vi "Example_OE2031&OE2041 Trig in.vi"() -> ()   [LabVIEW 2011]
panel:
  out "data_buffer":dbl[][](array[numeric])
  out "loss count":i32=-1
  out "cnt":u16
  in  "Ref_Source":u8(ring) items=["External", "Internal"]
  in  "Interval Count":u32=1 min=1 max=100000
  in  "选项卡控件":enum32{"选项卡 "}(tab)
  in  "Sweep Mode":u16(ring) items=["Linear", "Log"]
  in  "Start Frequency(Hz)":dbl=1000.0 min=1e-05 max=60000000.0 format="%#.3f"
  in  "Stop Frequency(Hz)":dbl=5000.0 min=1e-05 max=60000000.0 format="%#.3f"
  in  "Linear Step Frequency(Hz)":dbl=1000.0 min=1e-05 max=60000000.0 format="%#.3f"
  in  "Log Step Percent(%)":dbl=10.0 min=-100.0 max=100.0 format="%#.2f"
  in  "Step Time(ms)":i32=1000 min=50 max=100000
  in  "Sweep Run Mode":u16(ring) items=["Stop", "Singal", "Loop"]
  out "Group":u32
  in  "Sweep":u16(ring) items=["OFF", "ON"]
  in  "function":T1(ring)
  in  "Parameter Index":u16(ring) items=["X", "Y", "R", "θ", "Frequency", "XD1", "YD1", "RD1", "θD1", "XD2", "YD2", "RD2", "θD2", "XD3", "YD3", "RD3", "θD3", "X_Noise", "Y_Noise", "AUXADC1", "AUXADC2", "AUXADC3", "AUXADC4"]
  out "Wave":dbl(graph)
  in  "IP Address":string="192.168.1.10"
  in  "Timeout":u32=100
  in  "Port":u32=10001
  in  "Connect":bool
  in  "Trig Mode":u8(ring) items=["Internal", "Ext_Rissing_Edge", "Ext_Falling_Edge", "Ext_High_Level", "Ext_Low_Level"]
  out "Error out":errorcluster caption="error out"
  in  "Remote Mode":u16(ring) items=["USB"=0, "Ethernet"=3]
  in  "VISA resource name":refnum<visa-resource-name>
  # "Tel          :   +86-020-84133345\nWebsite  :   www.ssi-instrument.com\nE-mail     :   support@si-instrument.com"
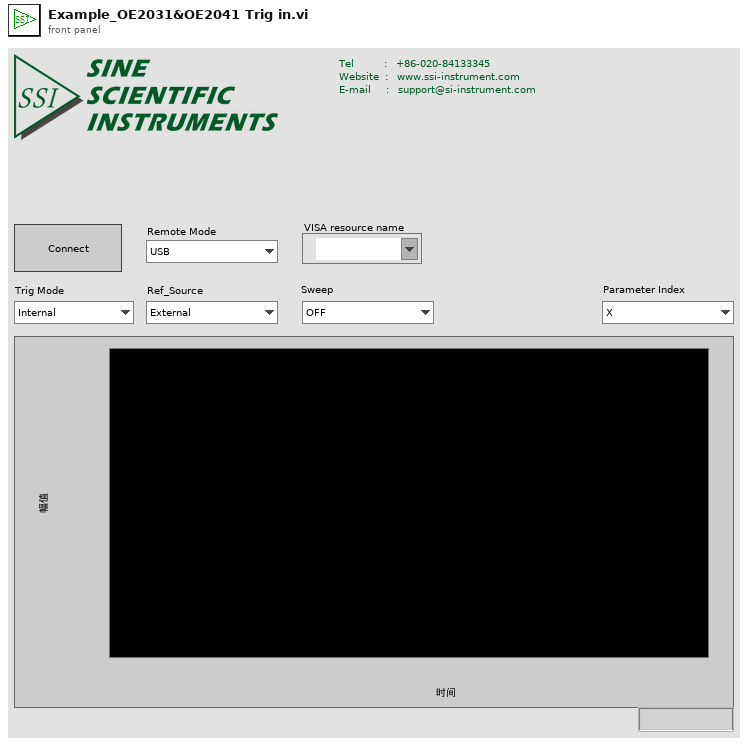
[diagram p1: front panel]
types:
  T1 = enum16{"initial", "Trig In Type", "Sample", "Ext_Sweep_Trig In", "Int_Sweep_Trig In"}
  T2 = enum8{"Enabled", "Disabled", "Disabled and Grayed Out"}
  T3 = cluster{"Port":u32, "Timeout":u32, "IP Address":string}
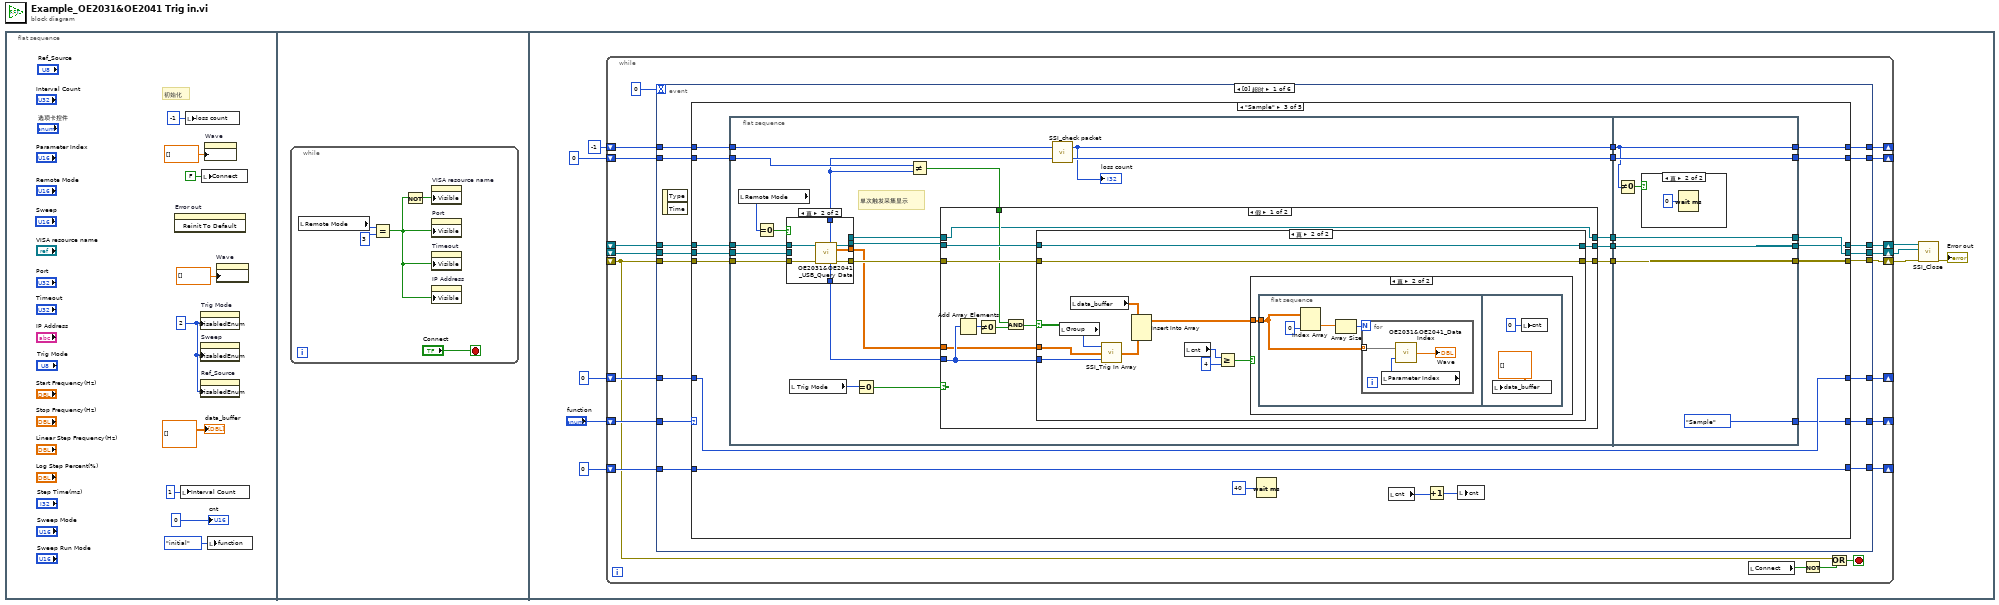
[diagram p0: block diagram]
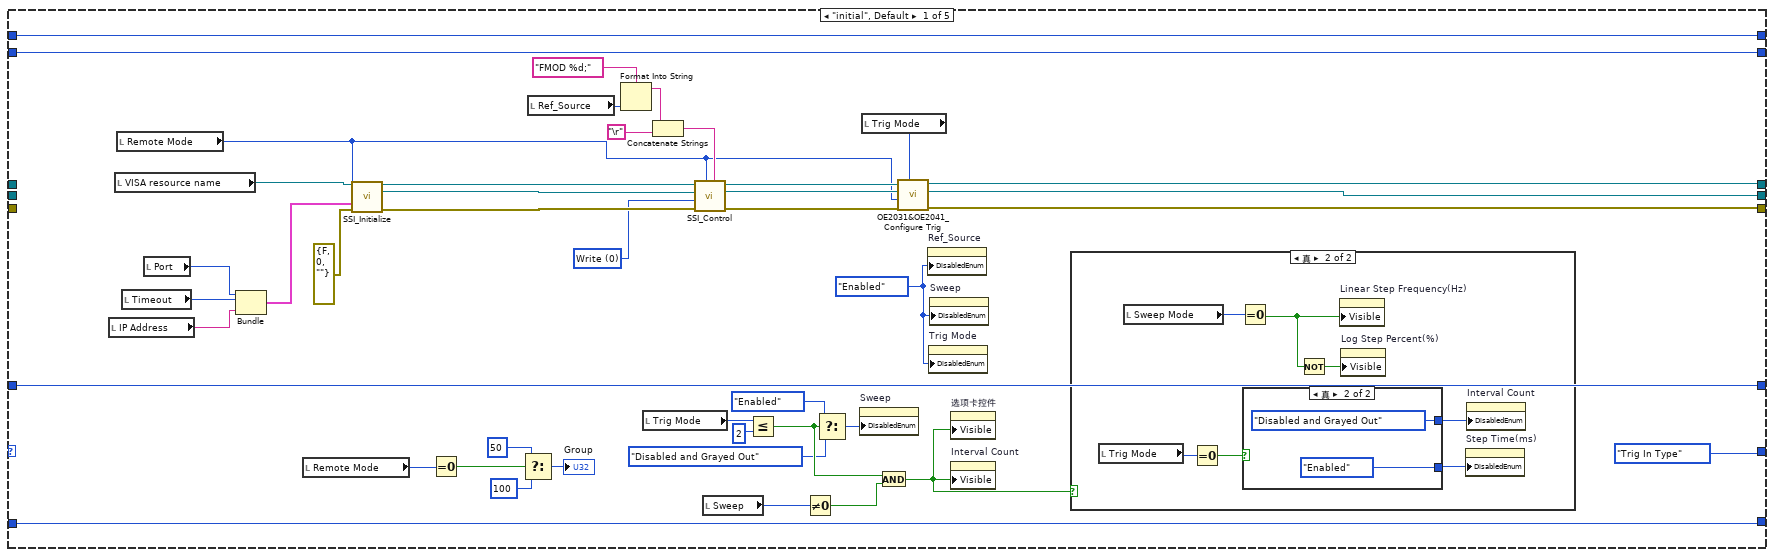
[diagram p2: hidden frame]
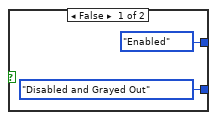
[diagram p4: hidden frame]
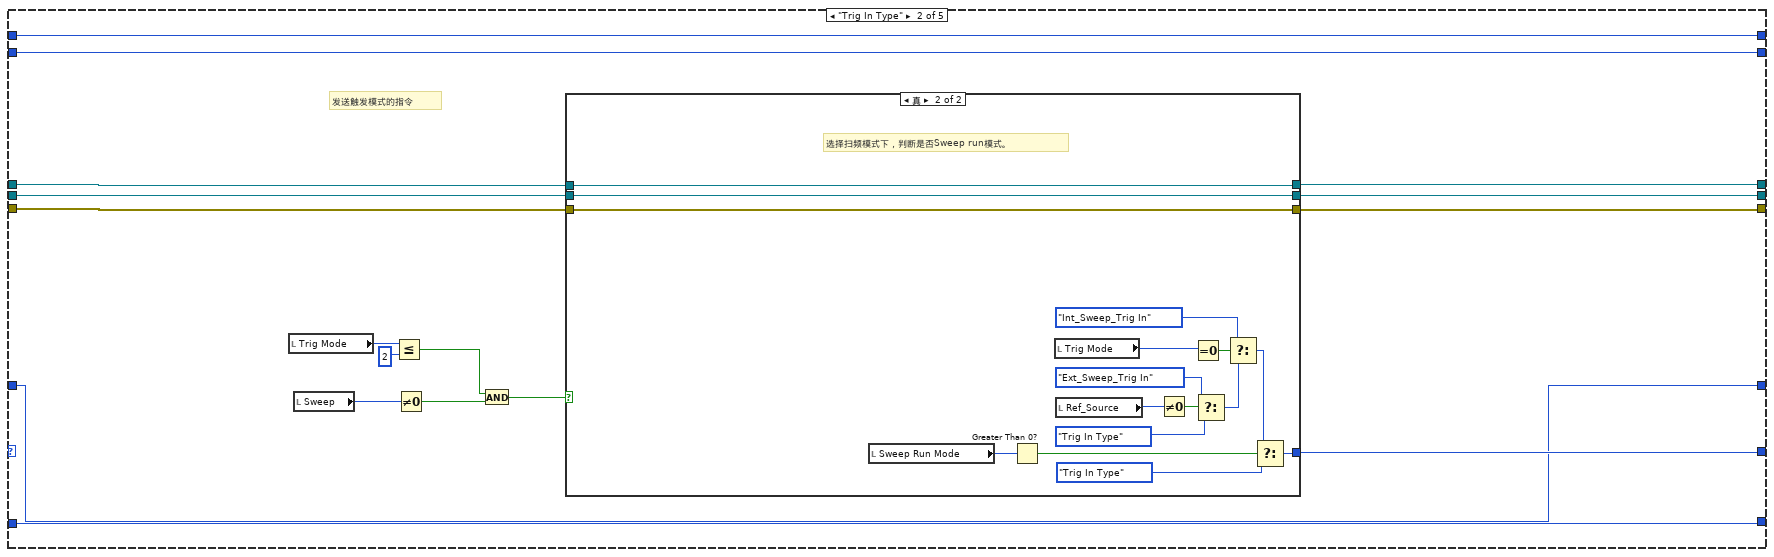
[diagram p5: hidden frame]
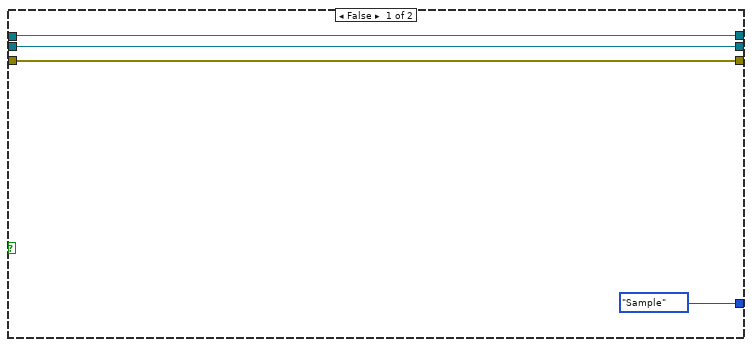
[diagram p6: hidden frame]
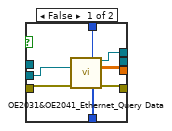
[diagram p7: hidden frame]
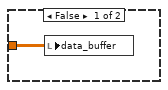
[diagram p9: hidden frame]
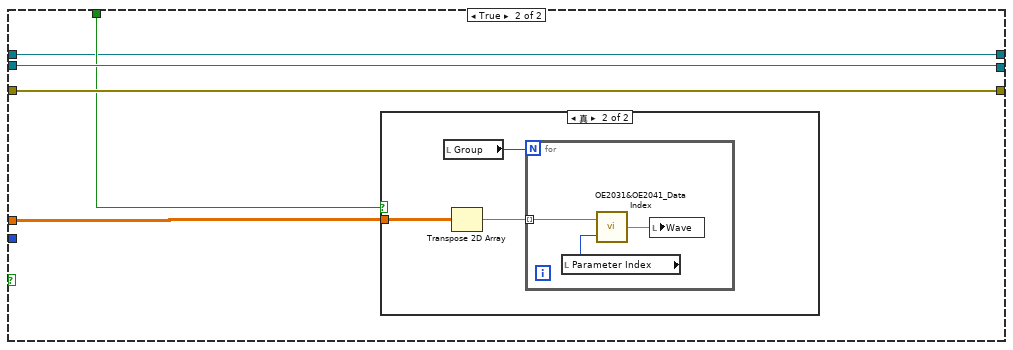
[diagram p10: hidden frame]
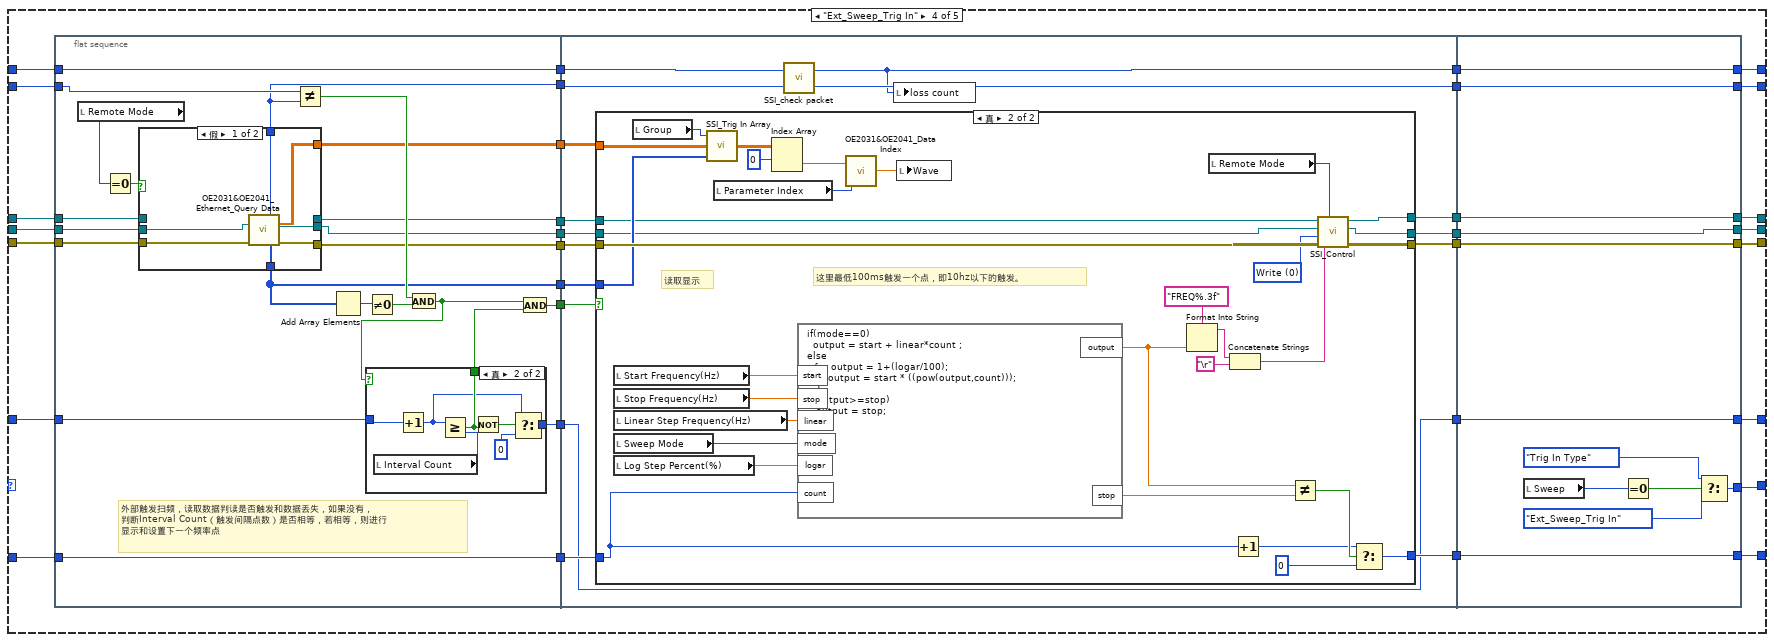
[diagram p13: hidden frame]
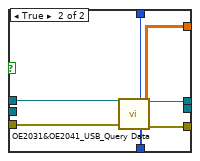
[diagram p14: hidden frame]
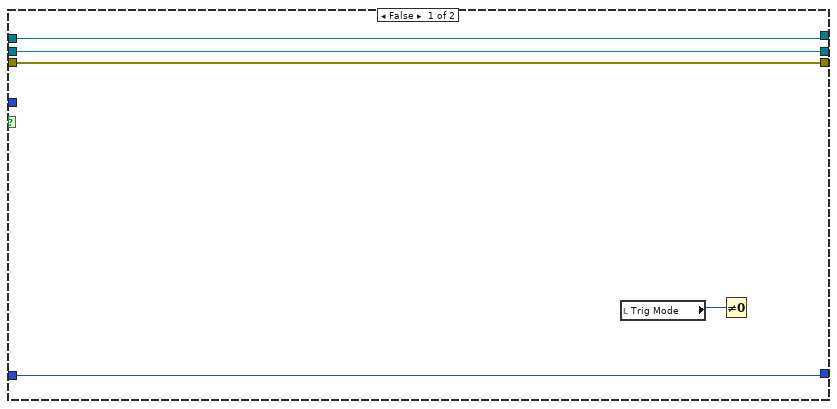
[diagram p16: hidden frame]
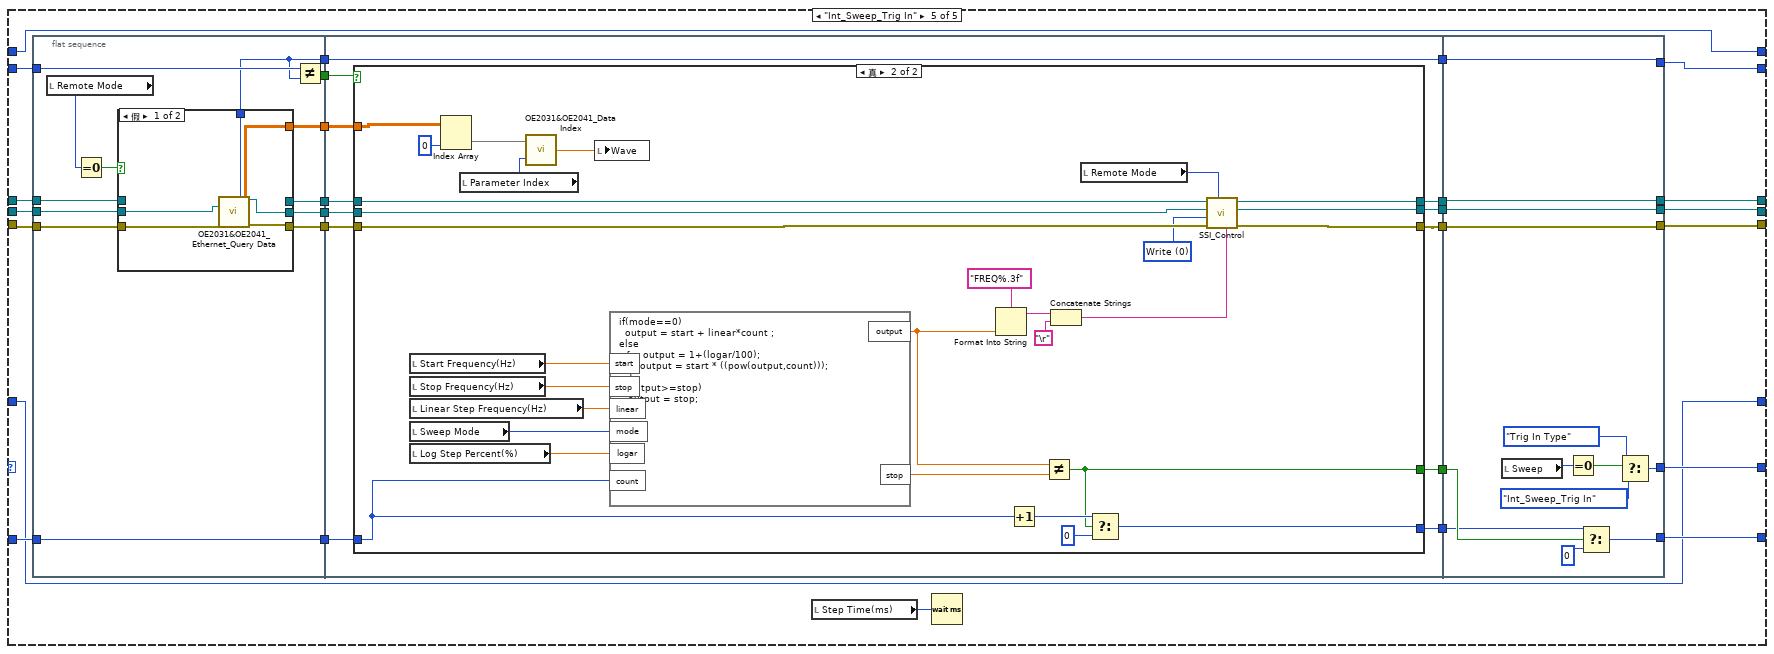
[diagram p17: hidden frame]
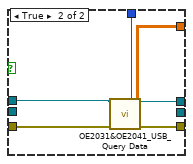
[diagram p18: hidden frame]
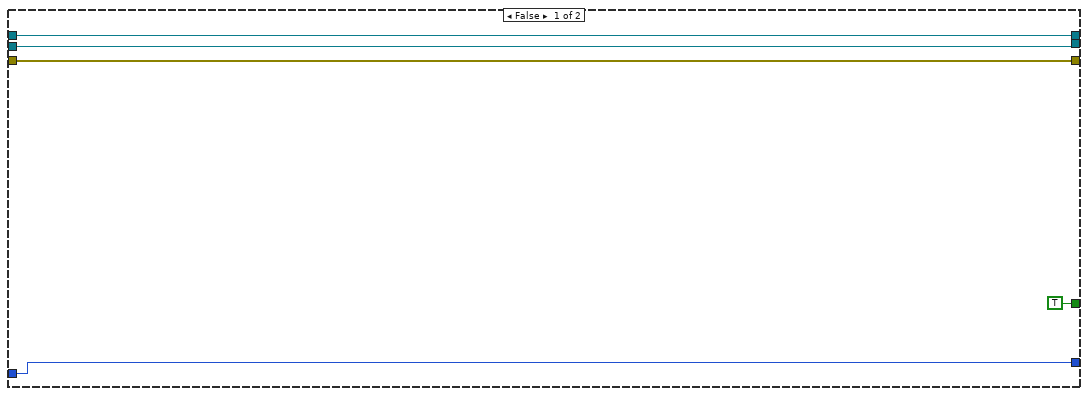
[diagram p19: hidden frame]
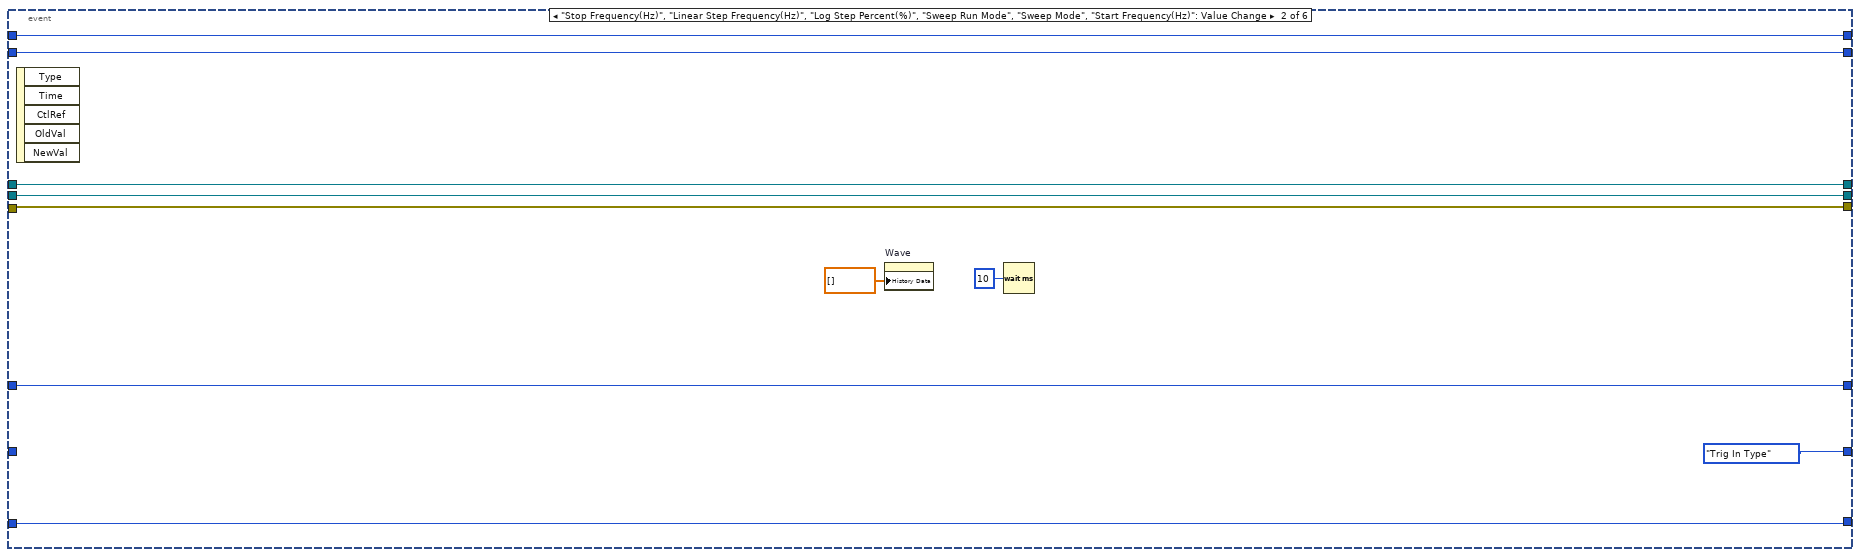
[diagram p20: hidden frame]
diagram:
  n1 = flat-sequence {
    frame #0 {
      w2 = 2
      # "初始化"
      n2 = invoke on="Error out" class="Clust (严格)" method="Reinit To Default"() -> ()  [unwired: 3 in, 3 out]
      n3 = local write "Interval Count"(u32 1 ("Interval Count")) -> ()
      n4 = local write "loss count"(-1 ("loss count")) -> ()
      n5 = property on="Trig Mode" class="Ring (严格)"("DisabledEnum"=w2) -> ()  [unwired: 2 in, 2 out]
      n6 = property on="Sweep" class="Ring (严格)"("DisabledEnum"=w2) -> ()  [unwired: 2 in, 2 out]
      n7 = property on="Ref_Source" class="Ring (严格)"("DisabledEnum"=w2) -> ()  [unwired: 2 in, 2 out]
      n8 = local write "Connect"(FALSE ("Connect")) -> ()
      n9 = property on="Wave" class="WFChart (严格)"("History Data"=dbl[] [] ("历史数据")) -> ()  [unwired: 2 in, 2 out]
      n10 = local write "function"(T1."initial" ("function")) -> ()
      n11 = property on="Wave" class="WFChart (严格)"("History Data"=dbl[] [] ("历史数据")) -> ()  [unwired: 2 in, 2 out]
      "data_buffer" <- dbl[][] []
      "cnt" <- 0
    }
    frame #1 {
      n12 = while {
        stop <- "Connect" stop-if-true
        n13 = local read "Remote Mode"() -> (w13:u16)
        n14 = Equal?(x=w13, y=u16 3) -> (x = y?=w11:bool)
        n15 = Not(x=w11) -> (.not. x?=w10:bool)
        n16 = property on="VISA resource name" class="VISAName"("Visible"=w10) -> ()  [unwired: 2 in, 2 out]
        n17 = property on="Port" class="DigNum (严格)"("Visible"=w11) -> ()  [unwired: 2 in, 2 out]
        n18 = property on="Timeout" class="DigNum (严格)"("Visible"=w11) -> ()  [unwired: 2 in, 2 out]
        n19 = property on="IP Address" class="Str"("Visible"=w11) -> ()  [unwired: 2 in, 2 out]
      }
    }
    frame #2 {
      n20 = while {
        shift-right: [w38] -> _
        shift-left: "function" -> [w39]
        shift-right: [w36] -> _
        shift-left: 0 ("f") -> [w37]
        shift-right: [w33] -> _
        shift-left: 0 -> [w34]
        shift-right: [w30] -> _
        shift-left: 0 -> [w31]
        shift-right: [w27] -> w17
        shift-left: _ -> [w41]
        shift-right: [w40] -> w22
        shift-left: _ -> [w29]
        shift-right: [w28] -> w18
        shift-left: _ -> [w26]
        shift-right: [w24] -> _
        shift-left: -1 ("loss count") -> [w25]
        stop <- w42 stop-if-true
        n21 = event shown="[0] 超时" {
          selector: _ -> [_ _ _ _ _ _]
          dyn-events: _ -> [_ _ _ _ _ _]
          timeout: 0 -> [_ _ _ _ _ _]
          tunnel: w41 -> [w59 w516 w528 w547 w573 w592]
          tunnel: [w58 w516 w528 w542 w572 w592] -> w27
          tunnel: [w57 w514 w527 w544 w575 w593] -> w40
          tunnel: w29 -> [w56 w514 w527 w549 w576 w593]
          tunnel: w39 -> [w55 _ _ _ w579 _]
          tunnel: [w54 T1."Trig In Type" ("function") T1."Trig In Type" ("function") T1."Trig In Type" ("function") w579 T1."Trig In Type" ("function")] -> w38
          tunnel: w37 -> [w53 w520 w530 w554 w580 w588]
          tunnel: [w52 w520 w530 w554 w580 w588] -> w36
          tunnel: w34 -> [w51 w518 w525 w552 w577 w590]
          tunnel: [w50 w518 w525 w552 w577 w590] -> w33
          tunnel: w31 -> [w49 w511 w524 w553 w578 w587]
          tunnel: [w48 w511 w524 w553 w578 w587] -> w30
          tunnel: [w47 w515 w522 w543 w571 w591] -> w28
          tunnel: w26 -> [w46 w515 w522 w548 w574 w591]
          tunnel: w25 -> [w45 w517 w521 w531 w566 w589]
          tunnel: [w44 w517 w521 w531 w566 w589] -> w24
          event Timeout {
            n22 = event-data() -> ()  [unwired: 1 in, 2 out]
            n23 = case shown="\"Sample\"" w55 {
              tunnel: w59 -> [_ w130 w170 w291 w411]
              tunnel: w56 -> [_ w128 w169 w290 w410]
              tunnel: [w81 w129 w153 w287 w424] -> w58
              tunnel: [w79 w127 w161 w288 w423] -> w57
              tunnel: [T1."Trig In Type" ("function") w126 w167 w276 w421] -> w54
              tunnel: w53 -> [w96 w125 w171 w289 w422]
              tunnel: [w96 w125 w171 w286 w420] -> w52
              tunnel: w51 -> [w94 w124 w166 w285 w426]
              tunnel: [w94 w124 w164 w284 w425] -> w50
              tunnel: w49 -> [w95 w123 w168 w271 w419]
              tunnel: [w95 w123 w168 w268 w419] -> w48
              tunnel: [w80 w115 w154 w264 w402] -> w47
              tunnel: w46 -> [_ w116 w156 w267 w406]
              tunnel: w45 -> [w61 w114 w159 w263 w401]
              tunnel: [w61 w114 w152 w260 w401] -> w44
              frame "initial", Default {
                w60 = T2."Enabled" ("禁用")
                w73 = u16 0 items=["Write", "Read"] ("Control")
                n24 = local read "IP Address"() -> (w76:string)
                n25 = local read "VISA resource name"() -> (w82:refnum<visa-resource-name>)
                n26 = local read "Remote Mode"() -> (w62:u16)
                n27 = local read "Timeout"() -> (w77:u32)
                n28 = local read "Port"() -> (w78:u32)
                n29 = Bundle("Port"=w78, "Timeout"=w77, "IP Address"=w76) -> (w75:T3)  [unwired: 1 in]
                n30 = local read "Remote Mode"() -> (w102:u16)
                n31 = call "SSI_Initialize.vi"("VISA resource name"=w82, "Remote Mode"=w62, "Ethernet"=w75, "error in (no error)"=errorcluster {"status"=FALSE, "code"=0, "source"=""}) -> ("VISA resource name out"=w86:refnum<visa-resource-name>, "connection ID(Ethernet)"=w87:refnum<k5>, "error out"=w83:errorcluster)  [unwired: 9 in]
                n32 = Equal To 0?(x=w102) -> (x = 0?=w98:bool)
                n33 = Select(t=50, s=w98, f=100) -> (s? t:f=→"Group":i32)
                n34 = local read "Ref_Source"() -> (w92:u8)
                n35 = Format Into String(format string="FMOD %d;" ("格式字符串"), w92) -> (resulting string=w93:string)  [unwired: 2 in, 1 out]
                n36 = local read "Trig Mode"() -> (w68:u8)
                n37 = Concatenate Strings(w93, "\r") -> (w72:string)
                n38 = call "SSI_Control.vi"("Write Buffer"=w72, "Remote Mode"=w62, "Error in (no error)"=w83, "Control"=w73, "Connection ID in"=w87, "VISA resource name"=w86) -> ("Error out"=w84:errorcluster, "Connection ID out"=w85:refnum<k5>, "VISA resource  out"=w88:refnum<visa-resource-name>)  [unwired: 2 in, 1 out]
                n39 = local read "Sweep"() -> (w69:u16)
                n40 = Less Or Equal?(x=w68, y=u8 2) -> (x <= y?=w70:bool)
                n41 = Not Equal To 0?(x=w69) -> (x != 0?=w71:bool)
                n42 = Select(t=T2."Enabled" ("禁用"), s=w70, f=T2."Disabled and Grayed Out") -> (s? t:f=w65:T2)
                n43 = property on="Sweep" class="Ring (严格)"("DisabledEnum"=w65) -> ()  [unwired: 2 in, 2 out]
                n44 = local read "Trig Mode"() -> (w89:u8)
                n45 = And(x=w70, y=w71) -> (x .and. y?=w63:bool)
                n46 = call "OE2031&OE2041_Configure Trig.vi"("Trig Mode"=w89, "Error in (no error)"=w84, "Remote Mode"=w62, "Connection ID in"=w85, "VISA resource name"=w88) -> ("Error out"=w79:errorcluster, "Connection ID out"=w80:refnum<k5>, "VISA resource  out"=w81:refnum<visa-resource-name>)  [unwired: 3 in, 1 out]
                n47 = property on="Ref_Source" class="Ring (严格)"("DisabledEnum"=w60) -> ()  [unwired: 2 in, 2 out]
                n48 = property on="Trig Mode" class="Ring (严格)"("DisabledEnum"=w60) -> ()  [unwired: 2 in, 2 out]
                n49 = property on="Sweep" class="Ring (严格)"("DisabledEnum"=w60) -> ()  [unwired: 2 in, 2 out]
                n50 = property on="选项卡控件" class="TabCtl (严格)"("Visible"=w63) -> ()  [unwired: 2 in, 2 out]
                n51 = property on="Interval Count" class="DigNum (严格)"("Visible"=w63) -> ()  [unwired: 2 in, 2 out]
                n52 = case shown="真" w63 {
                  frame False {
                  }
                  frame True {
                    n53 = local read "Trig Mode"() -> (w103:u8)
                    n54 = local read "Sweep Mode"() -> (w108:u16)
                    n55 = Equal To 0?(x=w103) -> (x = 0?=w104:bool)
                    n56 = Equal To 0?(x=w108) -> (x = 0?=w109:bool)
                    n57 = case shown="真" w104 {
                      tunnel: [T2."Disabled and Grayed Out" ("禁用") T2."Enabled" ("禁用")] -> w106
                      tunnel: [T2."Enabled" ("禁用") T2."Disabled and Grayed Out" ("禁用")] -> w105
                      frame False {
                      }
                      frame True {
                      }
                    }
                    n58 = Not(x=w109) -> (.not. x?=w107:bool)
                    n59 = property on="Linear Step Frequency(Hz)" class="DigNum (严格)"("Visible"=w109) -> ()  [unwired: 2 in, 2 out]
                    n60 = property on="Log Step Percent(%)" class="DigNum (严格)"("Visible"=w107) -> ()  [unwired: 2 in, 2 out]
                    n61 = property on="Step Time(ms)" class="DigNum (严格)"("DisabledEnum"=w106) -> ()  [unwired: 2 in, 2 out]
                    n62 = property on="Interval Count" class="DigNum (严格)"("DisabledEnum"=w105) -> ()  [unwired: 2 in, 2 out]
                  }
                }
              }
              frame "Trig In Type" {
                # "发送触发模式的指令"
                n63 = local read "Trig Mode"() -> (w120:u8)
                n64 = local read "Sweep"() -> (w119:u16)
                n65 = Less Or Equal?(x=w120, y=u8 2) -> (x <= y?=w118:bool)
                n66 = Not Equal To 0?(x=w119) -> (x != 0?=w117:bool)
                n67 = And(x=w118, y=w117) -> (x .and. y?=w122:bool)
                n68 = case shown="真" w122 {
                  tunnel: [w134 w146] -> w129
                  tunnel: [w133 w145] -> w127
                  tunnel: w128 -> [w133 w145]
                  tunnel: w130 -> [w134 w146]
                  tunnel: [T1."Sample" ("function") w149] -> w126
                  tunnel: w116 -> [w131 w135]
                  tunnel: [w131 w135] -> w115
                  frame False {
                  }
                  frame True {
                    # "选择扫频模式下，判断是否Sweep run模式。"
                    n69 = local read "Sweep Run Mode"() -> (w147:u16)
                    n70 = Greater Than 0?(x=w147) -> (x > 0?=w150:bool)
                    n71 = local read "Trig Mode"() -> (w140:u8)
                    n72 = local read "Ref_Source"() -> (w144:u8)
                    n73 = Not Equal To 0?(x=w144) -> (x != 0?=w143:bool)
                    n74 = Equal To 0?(x=w140) -> (x = 0?=w141:bool)
                    n75 = Select(t=T1."Ext_Sweep_Trig In" ("function"), s=w143, f=T1."Trig In Type" ("function")) -> (s? t:f=w142:T1)
                    n76 = Select(t=T1."Int_Sweep_Trig In" ("function"), s=w141, f=w142) -> (s? t:f=w148:T1)
                    n77 = Select(t=w148, s=w150, f=T1."Trig In Type" ("function")) -> (s? t:f=w149:T1)
                  }
                }
              }
              frame "Sample" {
                n78 = flat-sequence {
                  tunnel: w170 -> [w190]
                  tunnel: w169 -> [w189]
                  tunnel: w166 -> [w186]
                  tunnel: [w182] -> w165
                  tunnel: [w184] -> w163
                  tunnel: [w183] -> w162
                  tunnel: w159 -> [w181]
                  tunnel: w156 -> [w177]
                  tunnel: [w174] -> w155
                  tunnel: [w173] -> w151
                  tunnel: w165 -> [w253]
                  tunnel: w163 -> [w258]
                  tunnel: w162 -> [w257]
                  tunnel: [T1."Sample" ("function")] -> w167
                  tunnel: [w253] -> w164
                  tunnel: [w258] -> w153
                  tunnel: [w257] -> w161
                  tunnel: w155 -> [w255]
                  tunnel: [w255] -> w154
                  tunnel: [w252] -> w152
                  tunnel: w151 -> [w252]
                  frame #0 {
                    # "单次触发采集显示"
                    n79 = local read "Remote Mode"() -> (w178:u16)
                    n80 = Equal To 0?(x=w178) -> (x = 0?=w179:bool)
                    n81 = case shown="真" w179 {
                      tunnel: w190 -> [_ w205]
                      tunnel: w189 -> [w197 w204]
                      tunnel: [w194 w203] -> w187
                      tunnel: [w198 w202] -> w185
                      tunnel: [w193 w201] -> w182
                      tunnel: [w195 w200] -> w180
                      tunnel: w177 -> [w196 _]
                      tunnel: [_ w199] -> w176
                      tunnel: [w192 _] -> w175
                      frame False {
                        n82 = call "OE2031&OE2041_Ethernet_Query Data.vi"("Connection ID in"=w196, "Error in (no error)"=w197) -> ("Buffer Count"=w193:u8, "Connection ID out"=w192:refnum<k5>, "Total Data Array"=w195:dbl[][], "Trig In_Count"=w194:u8[], "Error out"=w198:errorcluster)  [unwired: 6 in, 3 out]
                      }
                      frame True {
                        n83 = call "OE2031&OE2041_USB_Query Data.vi"("VISA resource name"=w205, "Error in (no error)"=w204) -> ("Buffer Count"=w201:u8, "VISA resource  out"=w199:refnum<visa-resource-name>, "Total Data Array"=w200:dbl[][], "Trig In_Count"=w203:u8[], "Error out"=w202:errorcluster)  [unwired: 6 in, 3 out]
                      }
                    }
                    n84 = local read "Trig Mode"() -> (w191:u8)
                    n85 = Equal To 0?(x=w191) -> (x = 0?=w188:bool)
                    n86 = Not Equal?(x=w186, y=w182) -> (x != y?=w172:bool)
                    n87 = case shown="假" w188 {
                      tunnel: w180 -> [w208 w243]
                      tunnel: w187 -> [w215 _]
                      tunnel: w172 -> [w207 w242]
                      tunnel: w185 -> [w210 w244]
                      tunnel: w176 -> [w212 w245]
                      tunnel: [w211 w245] -> w184
                      tunnel: [w209 w244] -> w183
                      tunnel: w175 -> [w206 w241]
                      tunnel: [w206 w241] -> w174
                      frame False {
                        n88 = Add Array Elements(numeric array=w215) -> (sum=w216:u8)
                        n89 = Not Equal To 0?(x=w216) -> (x != 0?=w214:bool)
                        n90 = And(x=w207, y=w214) -> (x .and. y?=w213:bool)
                        n91 = case shown="真" w213 {
                          tunnel: w208 -> [_ w227]
                          tunnel: w215 -> [_ w226]
                          tunnel: [w218 w229] -> w211
                          tunnel: w212 -> [w218 w229]
                          tunnel: w210 -> [w217 w228]
                          tunnel: [w217 w228] -> w209
                          frame False {
                          }
                          frame True {
                            n92 = local read "Group"() -> (w225:u32)
                            n93 = local read "data_buffer"() -> (w224:dbl[][])
                            n94 = call "SSI_Trig In Array.vi"("Trig_Count"=w226, "Input Array"=w227, "Group"=w225) -> ("Output Array"=w223:dbl[][])
                            n95 = Insert Into Array(array=w224, new element=w223) -> (w222:dbl[][])  [unwired: 2 in]
                            n96 = local read "cnt"() -> (w221:u16)
                            n97 = Greater Or Equal?(x=w221, y=u16 4) -> (x >= y?=w219:bool)
                            n98 = case shown="真" w219 {
                              tunnel: w222 -> [w230 w231]
                              frame False {
                                n99 = local write "data_buffer"(w230) -> ()
                              }
                              frame True {
                                n100 = flat-sequence {
                                tunnel: w231 -> [w233]
                                frame #0 {
                                n101 = Index Array(array=w233, index (col)=0 ("禁用的索引 (列)")) -> (element=w232:dbl[])  [unwired: 1 in]
                                n102 = Array Size(array=w232) -> (size(s)=w235:i32)
                                n103 = for {
                                N: w235 -> [_]
                                tunnel: w233 -> [w236] mode=indexing
                                n104 = local read "Parameter Index"() -> (w238:u16)
                                n105 = call "OE2031&OE2041_Data Index.vi"("Parameter Type"=w238, "Input Date Array"=w236) -> ("Parameter"=→"Wave":dbl)
                                }
                                }
                                frame #1 {
                                n106 = local write "data_buffer"(dbl[][] [] ("data_buffer")) -> ()
                                n107 = local write "cnt"(u16 0 ("cnt")) -> ()
                                }
                                }
                              }
                            }
                          }
                        }
                      }
                      frame True {
                        n108 = case shown="真" w242 {
                          tunnel: w243 -> [_ w248]
                          frame False {
                          }
                          frame True {
                            n109 = local read "Group"() -> (w247:u32)
                            n110 = Transpose 2D Array(2D array=w248) -> (transposed array=w246:dbl[][])
                            n111 = for {
                              N: w247 -> [_]
                              tunnel: w246 -> [w250] mode=indexing
                              n112 = local read "Parameter Index"() -> (w251:u16)
                              n113 = call "OE2031&OE2041_Data Index.vi"("Parameter Type"=w251, "Input Date Array"=w250) -> ("Parameter"=w249:dbl)
                              n114 = local write "Wave"(w249) -> ()
                            }
                          }
                        }
                      }
                    }
                    n115 = call "SSI_check packet.vi"("input"=w182, "input loss"=w181) -> ("loss count"=w173:i32)  [unwired: 1 out]
                    "loss count" <- w173
                  }
                  frame #1 {
                    n116 = Not Equal To 0?(x=w252) -> (x != 0?=w254:bool)
                    n117 = case shown="真" w254 {
                      frame False {
                      }
                      frame True {
                        n118 = Wait (ms)(milliseconds to wait=u32 0 ("等待时间（毫秒）")) -> ()  [unwired: 1 out]
                      }
                    }
                  }
                }
                n119 = Wait (ms)(milliseconds to wait=40) -> ()  [unwired: 1 out]
                n120 = local read "cnt"() -> (w157:u16)
                n121 = Increment(x=w157) -> (x+1=w158:u16)
                n122 = local write "cnt"(w158) -> ()
              }
              frame "Ext_Sweep_Trig In" {
                n123 = flat-sequence {
                  tunnel: w291 -> [w312]
                  tunnel: w290 -> [w311]
                  tunnel: w289 -> [w309]
                  tunnel: [w305] -> w283
                  tunnel: w285 -> [w313]
                  tunnel: [w309] -> w282
                  tunnel: [w310] -> w281
                  tunnel: [w304] -> w275
                  tunnel: [w303] -> w274
                  tunnel: [w302] -> w273
                  tunnel: [w301] -> w272
                  tunnel: w271 -> [w299]
                  tunnel: [w297] -> w270
                  tunnel: w267 -> [w294]
                  tunnel: [w293] -> w266
                  tunnel: w263 -> [w292]
                  tunnel: [w292] -> w262
                  tunnel: w283 -> [w350]
                  tunnel: w281 -> [w337]
                  tunnel: w282 -> [w346]
                  tunnel: [w347] -> w280
                  tunnel: [w348] -> w279
                  tunnel: [w345] -> w278
                  tunnel: [w337] -> w277
                  tunnel: w275 -> [w349]
                  tunnel: w274 -> [w344]
                  tunnel: w273 -> [w343]
                  tunnel: w272 -> [w342]
                  tunnel: w270 -> [w341]
                  tunnel: [w341] -> w269
                  tunnel: w266 -> [w340]
                  tunnel: [w339] -> w265
                  tunnel: w262 -> [w338]
                  tunnel: [w336] -> w261
                  tunnel: [w398] -> w284
                  tunnel: [w399] -> w286
                  tunnel: [w396] -> w287
                  tunnel: [w397] -> w288
                  tunnel: w280 -> [w397]
                  tunnel: w279 -> [w396]
                  tunnel: w278 -> [w399]
                  tunnel: w277 -> [w398]
                  tunnel: [w394] -> w276
                  tunnel: w269 -> [w395]
                  tunnel: [w395] -> w268
                  tunnel: w265 -> [w389]
                  tunnel: [w389] -> w264
                  tunnel: w261 -> [w388]
                  tunnel: [w388] -> w260
                  frame #0 {
                    # "外部触发扫频，读取数据判读是否触发和数据丢失，如果没有，\n判断Interval Count（触发间隔点数）是否相等，若相等，则进行\n显示和设置下一个频率点"
                    n124 = local read "Remote Mode"() -> (w295:u16)
                    n125 = Equal To 0?(x=w295) -> (x = 0?=w296:bool)
                    n126 = case shown="假" w296 {
                      tunnel: w312 -> [_ w327]
                      tunnel: w311 -> [w320 w326]
                      tunnel: [w316 w325] -> w310
                      tunnel: [_ w324] -> w305
                      tunnel: [w319 w323] -> w304
                      tunnel: [w317 w322] -> w303
                      tunnel: [w315 w321] -> w302
                      tunnel: [w318 _] -> w293
                      tunnel: w294 -> [w314 _]
                      frame False {
                        n127 = call "OE2031&OE2041_Ethernet_Query Data.vi"("Connection ID in"=w314, "Error in (no error)"=w320) -> ("Buffer Count"=w316:u8, "Connection ID out"=w318:refnum<k5>, "Total Data Array"=w317:dbl[][], "Trig In_Count"=w315:u8[], "Error out"=w319:errorcluster)  [unwired: 6 in, 3 out]
                      }
                      frame True {
                        n128 = call "OE2031&OE2041_USB_Query Data.vi"("VISA resource name"=w327, "Error in (no error)"=w326) -> ("Buffer Count"=w325:u8, "VISA resource  out"=w324:refnum<visa-resource-name>, "Total Data Array"=w322:dbl[][], "Trig In_Count"=w321:u8[], "Error out"=w323:errorcluster)  [unwired: 6 in, 3 out]
                      }
                    }
                    n129 = Not Equal?(x=w313, y=w310) -> (x != y?=w307:bool)
                    n130 = Add Array Elements(numeric array=w302) -> (sum=w308:u8)
                    n131 = Not Equal To 0?(x=w308) -> (x != 0?=w306:bool)
                    n132 = And(x=w307, y=w306) -> (x .and. y?=w300:bool)
                    n133 = case shown="真" w300 {
                      tunnel: w299 -> [w328 w335]
                      tunnel: [_ w332] -> w298
                      tunnel: [w328 w329] -> w297
                      frame False {
                      }
                      frame True {
                        n134 = local read "Interval Count"() -> (w334:u32)
                        n135 = Increment(x=w335) -> (x+1=w331:i32)
                        n136 = Greater Or Equal?(x=w331, y=w334) -> (x >= y?=w332:bool)
                        n137 = Not(x=w332) -> (.not. x?=w333:bool)
                        n138 = Select(t=w331, s=w333, f=0) -> (s? t:f=w329:i32)
                      }
                    }
                    n139 = And(x=w300, y=w298) -> (x .and. y?=w301:bool)
                  }
                  frame #1 {
                    n140 = case shown="真" w342 {
                      tunnel: w349 -> [w354 w370]
                      tunnel: [w354 w372] -> w347
                      tunnel: [w355 w357] -> w348
                      tunnel: w350 -> [w355 w358]
                      tunnel: w346 -> [w353 w378]
                      tunnel: [w353 w377] -> w345
                      tunnel: w344 -> [_ w368]
                      tunnel: w343 -> [_ w366]
                      tunnel: w340 -> [w351 w362]
                      tunnel: [w351 w361] -> w339
                      frame False {
                        n141 = local read "Trig Mode"() -> (w352:u8)
                        n142 = Not Equal To 0?(x=w352) -> ()  [unwired: 1 out]
                      }
                      frame True {
                        w359 = u16 0 items=["Write", "Read"] ("Control")
                        # "这里最低100ms触发一个点，即10hz以下的触发。"
                        # "读取显示"
                        n143 = local read "Start Frequency(Hz)"() -> (w384:dbl)
                        n144 = local read "Stop Frequency(Hz)"() -> (w383:dbl)
                        n145 = local read "Linear Step Frequency(Hz)"() -> (w382:dbl)
                        n146 = local read "Sweep Mode"() -> (w381:u16)
                        n147 = local read "Log Step Percent(%)"() -> (w380:dbl)
                        n148 = local read "Group"() -> (w367:u32)
                        n149 = call "SSI_Trig In Array.vi"("Trig_Count"=w366, "Input Array"=w368, "Group"=w367) -> ("Output Array"=w365:dbl[][])
                        n150 = local read "Parameter Index"() -> (w369:u16)
                        n151 = Index Array(array=w365, index (row)=0 ("索引 (行)")) -> (element=w363:dbl[])  [unwired: 1 in]
                        n152 = formula code="if(mode==0)\n  output = start + linear*count ;\nelse \n  {    output = 1+(logar/100);\n       output = start * ((pow(output,count)));\n   }\nif(output>=stop)\n   output = stop;"("start"=w384, "stop"=w383, "linear"=w382, "logar"=w380, "mode"=w381, "count"=w378) -> ("stop"=w379:dbl, "output"=w373:dbl)
                        n153 = call "OE2031&OE2041_Data Index.vi"("Parameter Type"=w369, "Input Date Array"=w363) -> ("Parameter"=w364:dbl)
                        n154 = local write "Wave"(w364) -> ()
                        n155 = Format Into String(format string="FREQ%.3f" ("格式字符串"), w373) -> (resulting string=w386:string)  [unwired: 2 in, 1 out]
                        n156 = local read "Remote Mode"() -> (w360:u16)
                        n157 = Concatenate Strings(w386, "\r") -> (w371:string)
                        n158 = Increment(x=w378) -> (x+1=w375:i32)
                        n159 = Not Equal?(x=w373, y=w379) -> (x != y?=w376:bool)
                        n160 = call "SSI_Control.vi"("Write Buffer"=w371, "Remote Mode"=w360, "Error in (no error)"=w370, "Control"=w359, "Connection ID in"=w362, "VISA resource name"=w358) -> ("Error out"=w372:errorcluster, "Connection ID out"=w361:refnum<k5>, "VISA resource  out"=w357:refnum<visa-resource-name>)  [unwired: 2 in, 1 out]
                        n161 = Select(t=w375, s=w376, f=0) -> (s? t:f=w377:i32)
                      }
                    }
                    n162 = call "SSI_check packet.vi"("input"=w337, "input loss"=w338) -> ("loss count"=w336:i32)  [unwired: 1 out]
                    n163 = local write "loss count"(w336) -> ()
                  }
                  frame #2 {
                    n164 = local read "Sweep"() -> (w393:u16)
                    n165 = Equal To 0?(x=w393) -> (x = 0?=w392:bool)
                    n166 = Select(t=T1."Trig In Type" ("function"), s=w392, f=T1."Ext_Sweep_Trig In" ("function")) -> (s? t:f=w394:T1)
                  }
                }
              }
              frame "Int_Sweep_Trig In" {
                n167 = flat-sequence {
                  tunnel: [w436] -> w418
                  tunnel: [w431] -> w416
                  tunnel: [w435] -> w414
                  tunnel: w426 -> [w439]
                  tunnel: w422 -> [w437]
                  tunnel: w411 -> [w432]
                  tunnel: w410 -> [w434]
                  tunnel: [w438] -> w409
                  tunnel: [w437] -> w408
                  tunnel: w406 -> [w433]
                  tunnel: [w430] -> w405
                  tunnel: [w427] -> w404
                  tunnel: w418 -> [w463]
                  tunnel: [w463] -> w417
                  tunnel: w416 -> [w462]
                  tunnel: [w461] -> w415
                  tunnel: w414 -> [w460]
                  tunnel: [w459] -> w413
                  tunnel: [w455] -> w412
                  tunnel: w409 -> [w458]
                  tunnel: w408 -> [w457]
                  tunnel: [w456] -> w407
                  tunnel: w405 -> [w454]
                  tunnel: w404 -> [w453]
                  tunnel: [w452] -> w403
                  tunnel: [w510] -> w425
                  tunnel: w417 -> [w510]
                  tunnel: w415 -> [w509]
                  tunnel: [w509] -> w424
                  tunnel: [w508] -> w423
                  tunnel: w413 -> [w508]
                  tunnel: [w501] -> w421
                  tunnel: [w507] -> w420
                  tunnel: w412 -> [w505]
                  tunnel: w407 -> [w504]
                  tunnel: w403 -> [w498]
                  tunnel: [w498] -> w402
                  frame #0 {
                    n168 = local read "Remote Mode"() -> (w428:u16)
                    n169 = Equal To 0?(x=w428) -> (x = 0?=w429:bool)
                    n170 = case shown="假" w429 {
                      tunnel: [w443 w451] -> w436
                      tunnel: [_ w450] -> w431
                      tunnel: [w445 w449] -> w435
                      tunnel: [w444 w448] -> w430
                      tunnel: w434 -> [w442 w446]
                      tunnel: w433 -> [w441 _]
                      tunnel: w432 -> [_ w447]
                      tunnel: [w440 _] -> w427
                      frame False {
                        n171 = call "OE2031&OE2041_Ethernet_Query Data.vi"("Connection ID in"=w441, "Error in (no error)"=w442) -> ("Buffer Count"=w443:u8, "Connection ID out"=w440:refnum<k5>, "Total Data Array"=w444:dbl[][], "Error out"=w445:errorcluster)  [unwired: 6 in, 4 out]
                      }
                      frame True {
                        n172 = call "OE2031&OE2041_USB_Query Data.vi"("VISA resource name"=w447, "Error in (no error)"=w446) -> ("Buffer Count"=w451:u8, "VISA resource  out"=w450:refnum<visa-resource-name>, "Total Data Array"=w448:dbl[][], "Error out"=w449:errorcluster)  [unwired: 6 in, 4 out]
                      }
                    }
                    n173 = Not Equal?(x=w439, y=w436) -> (x != y?=w438:bool)
                  }
                  frame #1 {
                    n174 = case shown="真" w458 {
                      tunnel: w462 -> [w468 w471]
                      tunnel: [w468 w470] -> w461
                      tunnel: [w467 w477] -> w459
                      tunnel: w460 -> [w467 w478]
                      tunnel: w457 -> [w466 w491]
                      tunnel: [w466 w485] -> w456
                      tunnel: [TRUE w486] -> w455
                      tunnel: w454 -> [_ w474]
                      tunnel: w453 -> [w464 w473]
                      tunnel: [w464 w469] -> w452
                      frame False {
                      }
                      frame True {
                        w472 = u16 0 items=["Write", "Read"] ("Control")
                        n175 = local read "Start Frequency(Hz)"() -> (w497:dbl)
                        n176 = local read "Stop Frequency(Hz)"() -> (w496:dbl)
                        n177 = local read "Linear Step Frequency(Hz)"() -> (w495:dbl)
                        n178 = local read "Sweep Mode"() -> (w494:u16)
                        n179 = local read "Log Step Percent(%)"() -> (w493:dbl)
                        n180 = Index Array(array=w474, index (col)=0 ("禁用的索引 (列)")) -> (element=w479:dbl[])  [unwired: 1 in]
                        n181 = local read "Parameter Index"() -> (w482:u16)
                        n182 = call "OE2031&OE2041_Data Index.vi"("Parameter Type"=w482, "Input Date Array"=w479) -> ("Parameter"=w481:dbl)
                        n183 = local write "Wave"(w481) -> ()
                        n184 = formula code="if(mode==0)\n  output = start + linear*count ;\nelse \n  {    output = 1+(logar/100);\n       output = start * ((pow(output,count)));\n   }\nif(output>=stop)\n   output = stop;"("start"=w497, "stop"=w496, "linear"=w495, "logar"=w493, "mode"=w494, "count"=w491) -> ("stop"=w487:dbl, "output"=w483:dbl)
                        n185 = Format Into String(format string="FREQ%.3f" ("格式字符串"), w483) -> (resulting string=w488:string)  [unwired: 2 in, 1 out]
                        n186 = Increment(x=w491) -> (x+1=w492:i32)
                        n187 = Not Equal?(x=w483, y=w487) -> (x != y?=w486:bool)
                        n188 = Concatenate Strings(w488, "\r") -> (w476:string)
                        n189 = local read "Remote Mode"() -> (w475:u16)
                        n190 = Select(t=w492, s=w486, f=0) -> (s? t:f=w485:i32)
                        n191 = call "SSI_Control.vi"("Write Buffer"=w476, "Remote Mode"=w475, "Error in (no error)"=w478, "Control"=w472, "Connection ID in"=w473, "VISA resource name"=w471) -> ("Error out"=w477:errorcluster, "Connection ID out"=w469:refnum<k5>, "VISA resource  out"=w470:refnum<visa-resource-name>)  [unwired: 2 in, 1 out]
                      }
                    }
                  }
                  frame #2 {
                    n192 = local read "Sweep"() -> (w503:u16)
                    n193 = Equal To 0?(x=w503) -> (x = 0?=w502:bool)
                    n194 = Select(t=w504, s=w505, f=u16 0) -> (s? t:f=w507:i32)
                    n195 = Select(t=T1."Trig In Type" ("function"), s=w502, f=T1."Int_Sweep_Trig In" ("function")) -> (s? t:f=w501:T1)
                  }
                }
                n196 = local read "Step Time(ms)"() -> (w400:i32)
                n197 = Wait (ms)(milliseconds to wait=w400) -> ()  [unwired: 1 out]
              }
            }
          }
          event "Stop Frequency(Hz)", "Linear Step Frequency(Hz)", "Log Step Percent(%)", "Sweep Run Mode", "Sweep Mode", "Start Frequency(Hz)": Value Change {
            n198 = event-data() -> ()  [unwired: 1 in, 5 out]
            n199 = property on="Wave" class="WFChart (严格)"("History Data"=dbl[] [] ("历史数据")) -> ()  [unwired: 2 in, 2 out]
            n200 = Wait (ms)(milliseconds to wait=u32 10 ("等待时间（毫秒）")) -> ()  [unwired: 1 out]
          }
          event "Parameter Index": Value Change {
            n201 = event-data() -> ()  [unwired: 1 in, 5 out]
            n202 = property on="Wave" class="WFChart (严格)"("History Data"=dbl[] [] ("历史数据")) -> ()  [unwired: 2 in, 2 out]
            n203 = Wait (ms)(milliseconds to wait=u32 10 ("等待时间（毫秒）")) -> ()  [unwired: 1 out]
          }
          event "Trig Mode": Value Change {
            n204 = event-data() -> ()  [unwired: 1 in, 5 out]
            n205 = local read "Trig Mode"() -> (w545:u8)
            n206 = local read "Remote Mode"() -> (w546:u16)
            n207 = call "OE2031&OE2041_Configure Trig.vi"("Trig Mode"=w545, "Error in (no error)"=w549, "Remote Mode"=w546, "Connection ID in"=w548, "VISA resource name"=w547) -> ("Error out"=w544:errorcluster, "Connection ID out"=w543:refnum<k5>, "VISA resource  out"=w542:refnum<visa-resource-name>)  [unwired: 3 in, 1 out]
            n208 = local read "Trig Mode"() -> (w537:u8)
            n209 = local read "Sweep"() -> (w533:u16)
            n210 = Less Or Equal?(x=w537, y=u8 2) -> (x <= y?=w536:bool)
            n211 = Select(t=T2."Enabled" ("禁用"), s=w536, f=T2."Disabled and Grayed Out") -> (s? t:f=w540:T2)
            n212 = property on="Wave" class="WFChart (严格)"("History Data"=dbl[] [] ("历史数据")) -> ()  [unwired: 2 in, 2 out]
            n213 = Not Equal To 0?(x=w533) -> (x != 0?=w532:bool)
            n214 = property on="Sweep" class="Ring (严格)"("DisabledEnum"=w540) -> ()  [unwired: 2 in, 2 out]
            n215 = And(x=w536, y=w532) -> (x .and. y?=w535:bool)
            n216 = Wait (ms)(milliseconds to wait=u32 10 ("等待时间（毫秒）")) -> ()  [unwired: 1 out]
            n217 = property on="选项卡控件" class="TabCtl (严格)"("Visible"=w535) -> ()  [unwired: 2 in, 2 out]
            n218 = property on="Interval Count" class="DigNum (严格)"("Visible"=w535) -> ()  [unwired: 2 in, 2 out]
            n219 = case shown="真" w535 {
              frame False {
              }
              frame True {
                n220 = local read "Trig Mode"() -> (w555:u8)
                n221 = local read "Sweep Mode"() -> (w560:u16)
                n222 = Equal To 0?(x=w555) -> (x = 0?=w556:bool)
                n223 = Equal To 0?(x=w560) -> (x = 0?=w561:bool)
                n224 = case shown="真" w556 {
                  tunnel: [T2."Disabled and Grayed Out" ("禁用") T2."Enabled" ("禁用")] -> w558
                  tunnel: [T2."Enabled" ("禁用") T2."Disabled and Grayed Out" ("禁用")] -> w557
                  frame False {
                  }
                  frame True {
                  }
                }
                n225 = Not(x=w561) -> (.not. x?=w559:bool)
                n226 = property on="Linear Step Frequency(Hz)" class="DigNum (严格)"("Visible"=w561) -> ()  [unwired: 2 in, 2 out]
                n227 = property on="Log Step Percent(%)" class="DigNum (严格)"("Visible"=w559) -> ()  [unwired: 2 in, 2 out]
                n228 = property on="Step Time(ms)" class="DigNum (严格)"("DisabledEnum"=w558) -> ()  [unwired: 2 in, 2 out]
                n229 = property on="Interval Count" class="DigNum (严格)"("DisabledEnum"=w557) -> ()  [unwired: 2 in, 2 out]
              }
            }
          }
          event "Ref_Source": Value Change {
            w584 = u16 0 items=["Write", "Read"] ("Control")
            n230 = event-data() -> ()  [unwired: 1 in, 5 out]
            n231 = local read "Remote Mode"() -> (w570:u16)
            n232 = local read "Ref_Source"() -> (w582:u8)
            n233 = Format Into String(format string="FMOD %d;" ("格式字符串"), w582) -> (resulting string=w581:string)  [unwired: 2 in, 1 out]
            n234 = Concatenate Strings(w581, "\r") -> (w585:string)
            n235 = property on="Wave" class="WFChart (严格)"("History Data"=dbl[] [] ("历史数据")) -> ()  [unwired: 2 in, 2 out]
            n236 = call "SSI_Control.vi"("Write Buffer"=w585, "Remote Mode"=w570, "Error in (no error)"=w576, "Control"=w584, "Connection ID in"=w574, "VISA resource name"=w573) -> ("Error out"=w575:errorcluster, "Connection ID out"=w571:refnum<k5>, "VISA resource  out"=w572:refnum<visa-resource-name>)  [unwired: 2 in, 1 out]
            n237 = Wait (ms)(milliseconds to wait=u32 10 ("等待时间（毫秒）")) -> ()  [unwired: 1 out]
          }
          event "Sweep": Value Change {
            n238 = event-data() -> ()  [unwired: 1 in, 5 out]
            n239 = local read "Sweep"() -> (w595:u16)
            n240 = Not Equal To 0?(x=w595) -> (x != 0?=w586:bool)
            n241 = case shown="真" w586 {
              frame False {
              }
              frame True {
                n242 = local read "Trig Mode"() -> (w597:u8)
                n243 = local read "Sweep Mode"() -> (w602:u16)
                n244 = Equal To 0?(x=w597) -> (x = 0?=w598:bool)
                n245 = Equal To 0?(x=w602) -> (x = 0?=w603:bool)
                n246 = case shown="真" w598 {
                  tunnel: [T2."Disabled and Grayed Out" ("禁用") T2."Enabled" ("禁用")] -> w600
                  tunnel: [T2."Enabled" ("禁用") T2."Disabled and Grayed Out" ("禁用")] -> w599
                  frame False {
                  }
                  frame True {
                  }
                }
                n247 = Not(x=w603) -> (.not. x?=w601:bool)
                n248 = property on="Linear Step Frequency(Hz)" class="DigNum (严格)"("Visible"=w603) -> ()  [unwired: 2 in, 2 out]
                n249 = property on="Log Step Percent(%)" class="DigNum (严格)"("Visible"=w601) -> ()  [unwired: 2 in, 2 out]
                n250 = property on="Step Time(ms)" class="DigNum (严格)"("DisabledEnum"=w600) -> ()  [unwired: 2 in, 2 out]
                n251 = property on="Interval Count" class="DigNum (严格)"("DisabledEnum"=w599) -> ()  [unwired: 2 in, 2 out]
              }
            }
            n252 = property on="选项卡控件" class="TabCtl (严格)"("Visible"=w586) -> ()  [unwired: 2 in, 2 out]
            n253 = property on="Interval Count" class="DigNum (严格)"("Visible"=w586) -> ()  [unwired: 2 in, 2 out]
            n254 = property on="Wave" class="WFChart (严格)"("History Data"=dbl[] [] ("历史数据")) -> ()  [unwired: 2 in, 2 out]
          }
        }
        n255 = local read "Connect"() -> (w32:bool)
        n256 = Not(x=w32) -> (.not. x?=w43:bool)
        n257 = Or(x=w29, y=w43) -> (x .or. y?=w42:bool)
      }
      n258 = call "SSI_Close.vi"("Error in (no error)"=w22, "Connection ID in"=w18, "VISA resource name"=w17) -> ("Error out"=→"Error out":errorcluster)  [unwired: 4 in]
    }
  }
